vi "Mask Write Register Response.vi"(8 "error in (no error)":errorcluster, 9 "Modbus Data Unit in":T1={"function"=1, "Data"=[]} {"function" items=["Read Discrete Inputs"=2, "Read Coils"=1, "Write Single Coil"=5, "Write Multiple Coils"=15, "Read Input Register"=4, "Read Holding Registers"=3, "Write Single Register"=6, "Write Multiple Registers"=16, "Read/Write Multiple Registers"=23, "Mask Write Register"=22, "Read FIFO Queue"=24, "Read File Record"=20, "Write File Record"=21, "Read Exception Status"=7, "Diagnostic"=8, "Get Com Event Counter"=11, "Get Com Event Log"=12, "Report Slave ID"=17, "Read Device Identification"=43]; "Data" format="%.0x"}) -> (0 "error out":errorcluster, 1 "AND mask":u16, 2 "address":u16, 5 "OR mask":u16)   [LabVIEW 2019, in "NI_modbus_upd.lvlib"]
doc: "Decodes the response for the masked write single register function."
uses:
  NI_modbus_upd.lvlib
  Ctl/MB Modbus Data Unit.ctl
  Modbus Data Unit (PDU)/Function.ctl
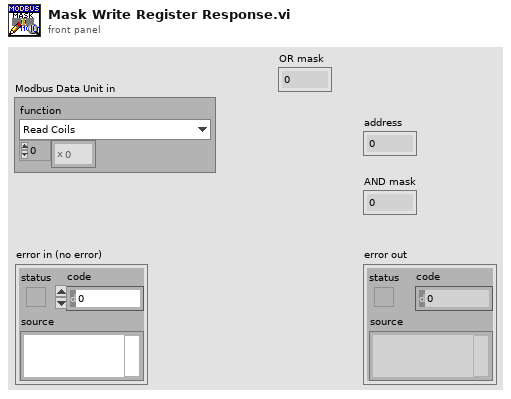
[diagram p1: front panel]
types:
  T1 = typedef "NI_modbus_upd.lvlib/MB Modbus Data Unit.ctl" = cluster{"function":T2, "Data":u8[]}
  T2 = typedef "NI_modbus_upd.lvlib/Function.ctl" = u8
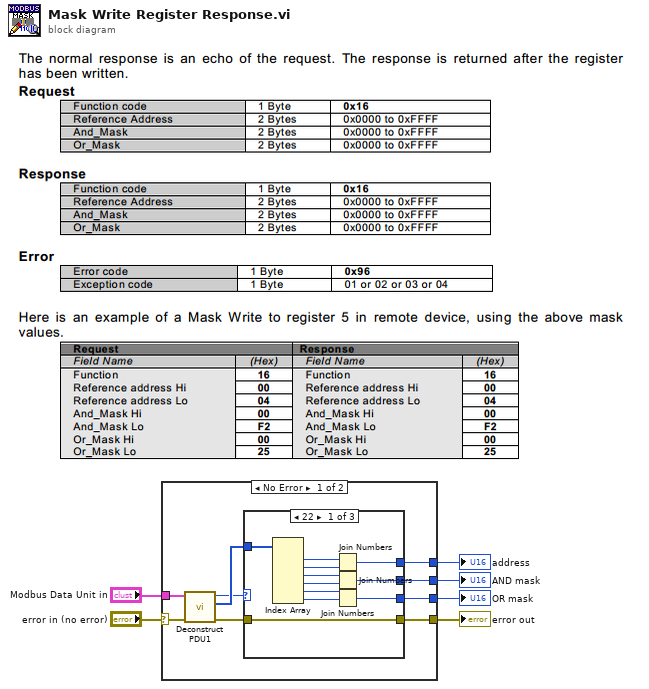
[diagram p0: block diagram]
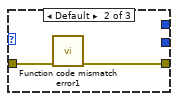
[diagram p2: hidden frame]
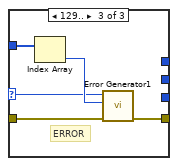
[diagram p3: hidden frame]
diagram:
  n1 = case shown="No Error" "error in (no error)" {
    selector: "error in (no error)" -> [w7 w34]
    tunnel: [w15 w34] -> w6
    tunnel: "Modbus Data Unit in" -> [w13 _]
    tunnel: [w11 _] -> w5
    tunnel: [w10 _] -> w4
    tunnel: [w8 _] -> w3
    frame No Error {
      n2 = call "Deconstruct PDU1.vi"("error in (no error)"=w7, "Modbus Data Unit in"=w13) -> ("error out"=w12:errorcluster, "data"=w14:u8[], "function"=w9:T2)  [unwired: 7 in]
      n3 = case shown="22" w9 {
        selector: w9 -> [_ _ w29]
        tunnel: w12 -> [w25 w27 w30]
        tunnel: w14 -> [w26 _ w33]
        tunnel: [w25 w28 w32] -> w15
        tunnel: [w24 _ _] -> w11
        tunnel: [w23 _ _] -> w10
        tunnel: [w16 _ _] -> w8
        frame 22 {
          n4 = Index Array(array=w26) -> (element #1=w22:u8, element #2=w21:u8, element #3=w20:u8, element #4=w19:u8, element #5=w18:u8, element #6=w17:u8)  [unwired: 6 in]
          n5 = Join Numbers(hi=w22, lo=w21) -> ((hi.lo)=w24:u16)
          n6 = Join Numbers(hi=w20, lo=w19) -> ((hi.lo)=w23:u16)
          n7 = Join Numbers(hi=w18, lo=w17) -> ((hi.lo)=w16:u16)
        }
        frame Default {
          n8 = call "Function code mismatch error1.vi"("error in (no error)"=w27) -> ("error out"=w28:errorcluster)  [unwired: 10 in]
        }
        frame 129.. {
          # "ERROR"
          n9 = Index Array(array=w33) -> (element=w31:u8)  [unwired: 1 in]
          n10 = call "Error Generator1.vi"("error in (no error)"=w30, "data return (error code)"=w31, "function return"=w29) -> ("error out"=w32:errorcluster)  [unwired: 8 in]
        }
      }
    }
    frame Error {
    }
  }
  "error out" <- w6
  "address" <- w5
  "AND mask" <- w4
  "OR mask" <- w3
